vi "process_2.vi"(6 "iteration number":i32, 8 "error in (no error)":errorcluster, 9 "# square points":i32, 10 "array in":u16[](array[numeric]), 11 "cluster in":T1={"reception"={"square size"=3, "offset"=0, "# squares out"=0, "left over"=[], "raps points length"=1}, "fft"={"reference"=[]}}) -> (0 "error out":errorcluster, 2 "offset found":i32[](array[numeric]), 3 "cluster out":T1={"reception"={"square size"=3, "offset"=0, "# squares out"=0, "left over"=[], "raps points length"=1}, "fft"={"reference"=[]}}, 5 "array found":dbl[][](array[numeric]))   [LabVIEW 2010]
uses:
  motion_correction_cluster.ctl
  <vilib>/Analysis/2dsp.llb/2D Real FFT.vi
  <vilib>/Analysis/2dsp.llb/2D Inverse Real FFT.vi
  <vilib>/Analysis/NI_AALPro.lvlib
  <vilib>/Analysis/2dsp.llb/2D Cross Correlation (DBL).vi
panel:
  out "Intensity Graph":dbl[][](graph)
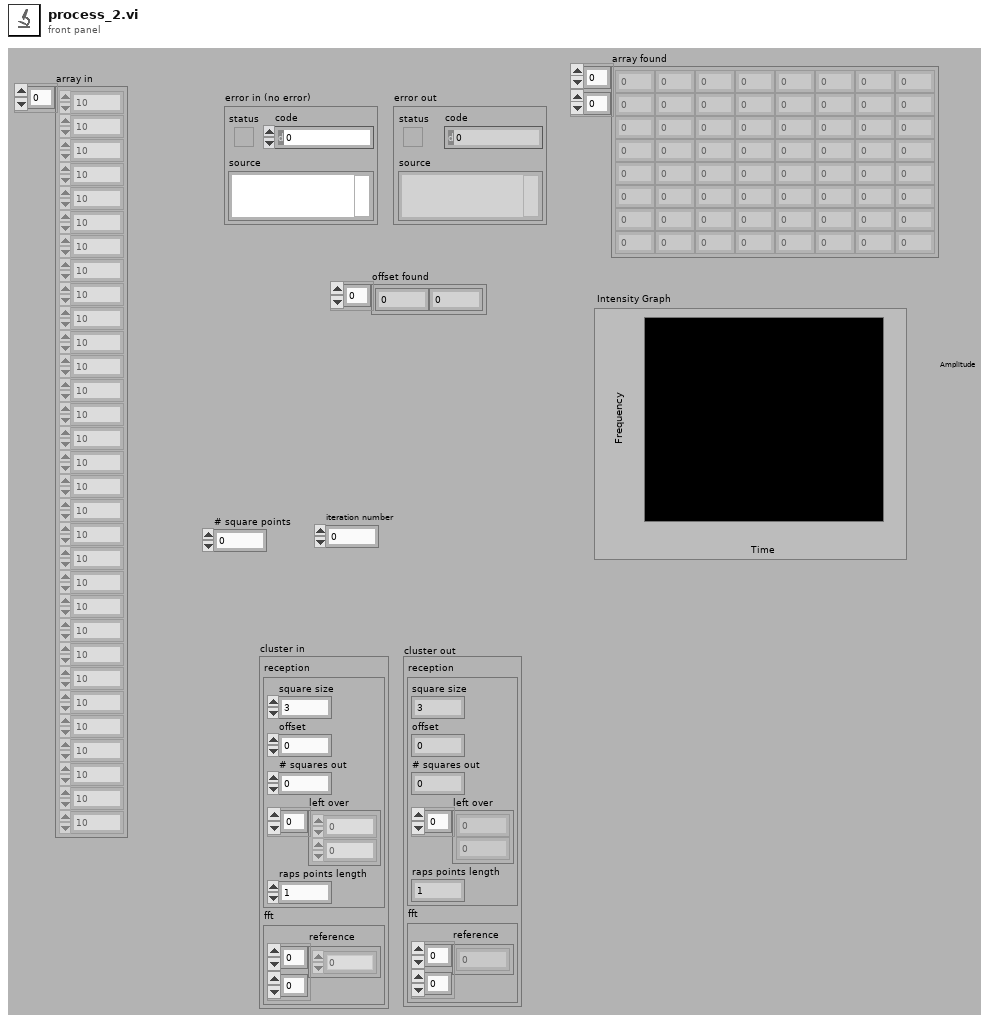
[diagram p1: front panel]
types:
  T1 = typedef "motion_correction_cluster.ctl" = cluster{"reception":cluster{"square size":i32, "offset":i32, "# squares out":i32, "left over":u16[], "raps points length":i32}, "fft":cluster{"reference":dbl[][]}}
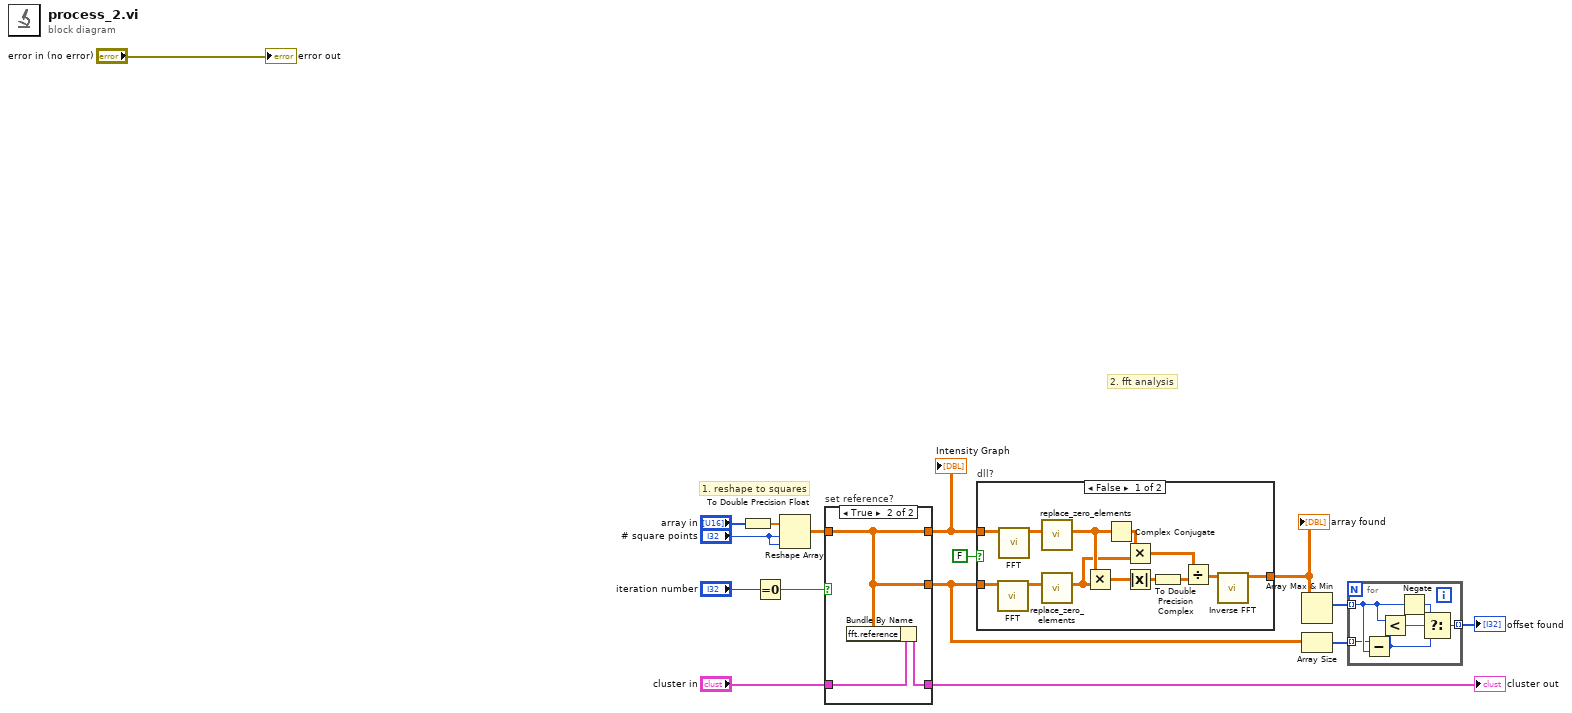
[diagram p0: block diagram]
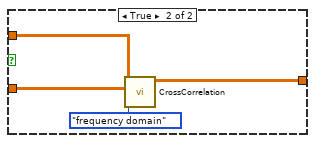
[diagram p2: hidden frame]
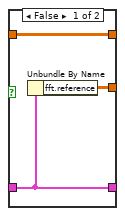
[diagram p3: hidden frame]
diagram:
  # "2. fft analysis"
  # "1. reshape to squares"
  n1 = To Double Precision Float(number="array in") -> (double precision float=w10:dbl[])
  n2 = Equal To 0?(x="iteration number") -> (x = 0?=w5:bool)
  n3 = Reshape Array(w10, "# square points", "# square points") -> (w4:dbl[][])
  n4 = case "set reference?" shown="True" w5 {
    tunnel: [w19 w22] -> w1
    tunnel: "cluster in" -> [w18 w21]
    tunnel: [w18 w20] -> w6
    tunnel: w4 -> [w17 w22]
    tunnel: [w17 w22] -> w3
    frame False {
      n5 = Unbundle By Name(w18) -> ("fft.reference"=w19:dbl[][])
    }
    frame True {
      n6 = Bundle By Name(cluster=w21, "fft.reference"=w22) -> (w20:T1)
    }
  }
  "cluster out" <- w6
  "Intensity Graph" <- w3
  n7 = case "dll?" shown="False" FALSE {
    tunnel: w1 -> [w35 w38]
    tunnel: [w34 w37] -> w15
    tunnel: w3 -> [w27 w39]
    frame False {
      n8 = call-poly <vilib>:"FFT.vi"("X"=w35) -> ("FFT {X}"=w24:cdb[][])  [unwired: 9 in, 1 out]
      n9 = call-poly <vilib>:"FFT.vi"("X"=w27) -> ("FFT {X}"=w26:cdb[][])  [unwired: 9 in, 1 out]
      n10 = call "replace_zero_elements.vi"("array in"=w26) -> ("array out"=w25:cdb[][])  [unwired: 10 in]
      n11 = call "replace_zero_elements.vi"("array in"=w24) -> ("array out"=w23:cdb[][])  [unwired: 10 in]
      n12 = Multiply(x=w25, y=w23) -> (x*y=w30:cdb[][])
      n13 = Complex Conjugate(1:w25) -> (0:w33:cdb[][])
      n14 = Multiply(x=w33, y=w23) -> (x*y=w31:cdb[][])
      n15 = Absolute Value(x=w30) -> (abs(x)=w29:dbl[][])
      n16 = To Double Precision Complex(1:w29) -> (0:w28:cdb[][])
      n17 = Divide(x=w31, y=w28) -> (x/y=w32:cdb[][])
      n18 = call-poly <vilib>:"Inverse FFT.vi"("FFT {X}"=w32) -> ("X"=w34:dbl[][])  [unwired: 9 in, 1 out]
    }
    frame True {
      n19 = call-poly <vilib>:"CrossCorrelation.vi"("algorithm"=enum32{"direct", "frequency domain"}."frequency domain", "Y"=w38, "X"=w39) -> ("Rxy"=w37:dbl[][])  [unwired: 7 in, 1 out]
    }
  }
  "array found" <- w15
  n20 = Array Max & Min(array=w15) -> (max index (indices)=w14:i32[])  [unwired: 3 out]
  n21 = Array Size(array=w1) -> (size(s)=w13:i32[])
  n22 = for {
    tunnel: w14 -> [w45] mode=indexing
    tunnel: w13 -> [w44] mode=indexing
    tunnel: [w40] -> w9 mode=indexing
    n23 = Subtract(x=w44, y=w45) -> (x-y=w43:i32)
    n24 = Less?(x=w45, y=w43) -> (x < y?=w41:bool)
    n25 = Negate(x=w45) -> (-x=w42:i32)
    n26 = Select(t=w42, s=w41, f=w43) -> (s? t:f=w40:i32)
  }
  "offset found" <- w9
  "error out" <- "error in (no error)"
